vi "Write variant to file.vi"(8 "error in (no error)":errorcluster, 9 "variant":variant, 10 "Group name":string, 11 "tdms file":refnum<k34>) -> (0 "error out":errorcluster, 3 "tdms file out":refnum<k34>)   [LabVIEW 2015]
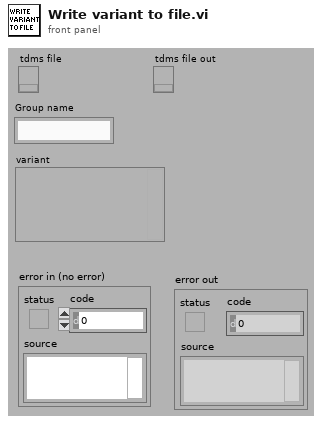
[diagram p1: front panel]
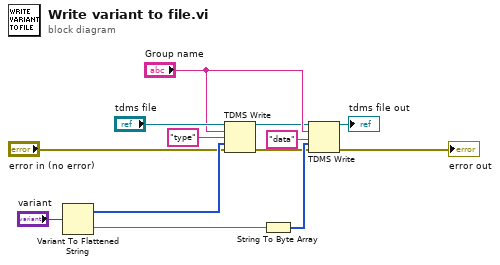
[diagram p0: block diagram]
diagram:
  n1 = Variant To Flattened String(Variant="variant") -> (data string=w11:string, 1:w8:i16[])
  n2 = TDMS Write(0:"tdms file", 5:"Group name", 7:"type", 9:w8, 11:"error in (no error)") -> (4:w3:refnum<k34>, 15:w10:errorcluster)  [unwired: 1 in, 2 out]
  n3 = String To Byte Array(string=w11) -> (unsigned byte array=w12:u8[])
  n4 = TDMS Write(0:w3, 5:"Group name", 7:"data", 9:w12, 11:w10) -> (4:→"tdms file out":refnum<k34>, 15:→"error out":errorcluster)  [unwired: 1 in, 2 out]
